vi "DSF.Engine.Interface.RT FIFO.Read.32B.vi"(7 "FIFO Debug Flags":refnum<class "DSF.Engine.Debug Flags.FIFO.lvclass">, 8 "error in (no error)":errorcluster, 9 "timeout in ms (0)":i32, 11 "RT FIFO in":T1) -> (0 "error out":errorcluster, 1 "empty?":bool, 2 "element out":T2, 3 "RT FIFO out":T1, 4 "# elements":u32)   [LabVIEW 2017, in "DSF.Engine.lvlib" / "DSF.Engine.Interface.lvclass"]
uses:
  DSF.Engine.Interface.lvclass
  DSF.Engine.Interface.RT FIFO.Data.32B.ctl
  DSF.Engine.Interface.RT FIFO.Payload.32B.ctl
  DSF.Engine.Interface.RT FIFO.Ref.32B.ctl
  Debug/DSF.Engine.Debug Flags.FIFO.lvclass
  Debug/DSF.Engine.Debug Flags.FIFO.lvclass/DSF.Engine.Debug Flags.FIFO.ctl
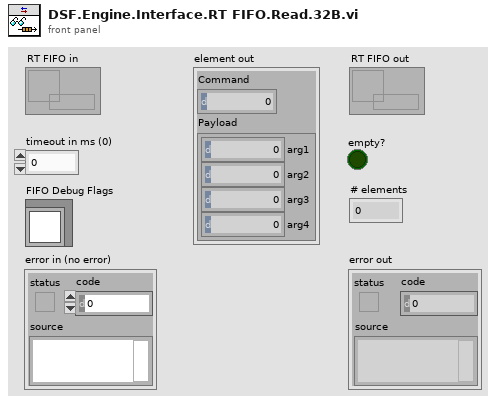
[diagram p1: front panel]
types:
  T1 = typedef "DSF.Engine.lvlib/DSF.Engine.Interface.lvclass/DSF.Engine.Interface.RT FIFO.Ref.32B.ctl" = refnum<k33>
  T2 = typedef "DSF.Engine.lvlib/DSF.Engine.Interface.lvclass/DSF.Engine.Interface.RT FIFO.Data.32B.ctl" = cluster{"Command":u8, "Payload":T3}
  T3 = typedef "DSF.Engine.lvlib/DSF.Engine.Interface.lvclass/DSF.Engine.Interface.RT FIFO.Payload.32B.ctl" = cluster{"arg1":u64, "arg2":u64, "arg3":u64, "arg4":u64}
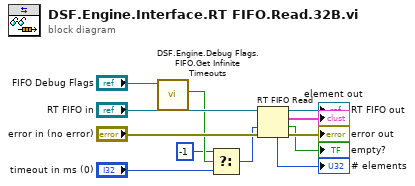
[diagram p0: block diagram]
diagram:
  n1 = call "DSF.Engine.Debug Flags.FIFO.Get Infinite Timeouts.vi"("FIFO Debug Flags in"="FIFO Debug Flags") -> ("infinite timeouts"=w5:bool)  [unwired: 9 in, 1 out]
  n2 = Select(t=-1, s=w5, f="timeout in ms (0)") -> (s? t:f=w2:i32)
  n3 = RT FIFO Read(0:"RT FIFO in", 2:w2, 3:"error in (no error)") -> (7:→"# elements":u32, 8:→"RT FIFO out":T1, 9:→"element out":T2, 10:→"empty?":bool, 11:→"error out":errorcluster)  [unwired: 1 in]
